vi "GetBounds.vi"(0 "ESC in":refnum<class "ESC.lvclass">, 11 "error in (no error)":errorcluster) -> (4 "ESC out":refnum<class "ESC.lvclass">, 10 "Calibrate?":bool, 12 "PWM Frequency":dbl, 13 "Duty Cycle Min":dbl, 14 "Duty Cycle Max":dbl, 15 "error out":errorcluster)   [LabVIEW 2015, in "ESC.lvclass"]
uses:
  ESC.lvclass
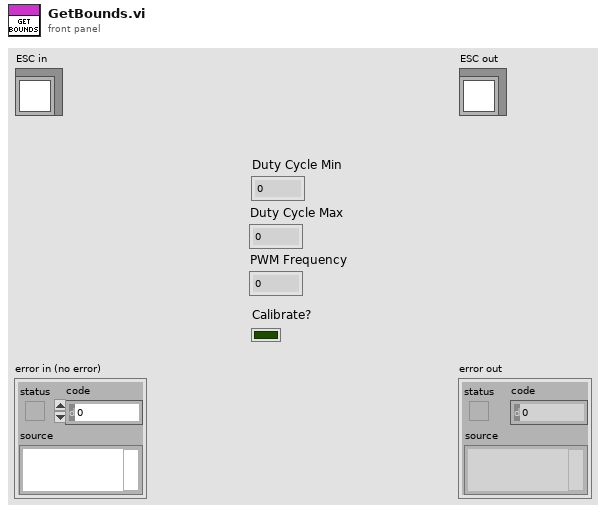
[diagram p1: front panel]
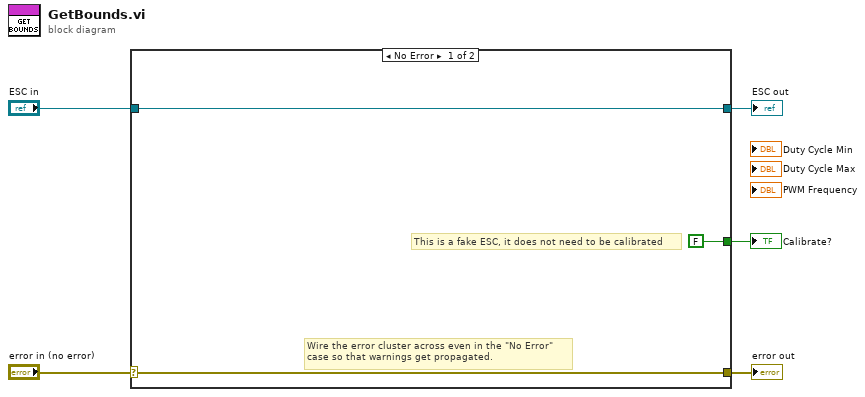
[diagram p0: block diagram]
diagram:
  n1 = case shown="No Error" "error in (no error)" {
    selector: "error in (no error)" -> [w7 w10]
    tunnel: [w7 w10] -> w4
    tunnel: [w8 w9] -> w2
    tunnel: "ESC in" -> [w8 w9]
    tunnel: [FALSE ("Calibrate?") _] -> w1
    frame No Error {
      # "This is a fake ESC, it does not need to be calibrated"
      # "Wire the error cluster across even in the \"No Error\"\ncase so that warnings get propagated."
    }
    frame Error {
    }
  }
  "error out" <- w4
  "ESC out" <- w2
  "Calibrate?" <- w1
